vi "TSM DAQmx Relay Initialize Sessions.vi"(0 "TSM context":T1) -> (15 "error out":errorcluster)   [LabVIEW 2019]
doc: "Use this VI to initialize sessions for all NI 2567 Relay Driver Instruments in the pin map associated with the test program."
uses:
  <vilib>/NI_TestStand_SemiconductorModule/NI_TestStand_Semiconductor_Module.lvlibp/PinMap/General/SemiconductorModuleContext.ctl
  <vilib>/DAQmx/create/channels.llb/DAQmx Create Channel (DO-Digital Output).vi
  <vilib>/NI_TestStand_SemiconductorModule/NI_TestStand_Semiconductor_Module.lvlibp
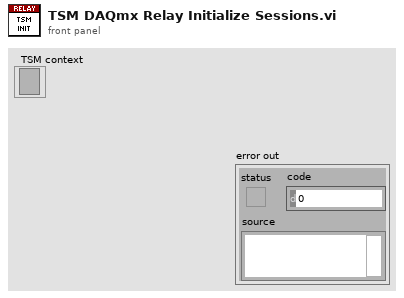
[diagram p1: front panel]
types:
  T1 = typedef "NI_TestStand_Semiconductor_Module.lvlibp/SemiconductorModuleContext.ctl" = refnum<k7>
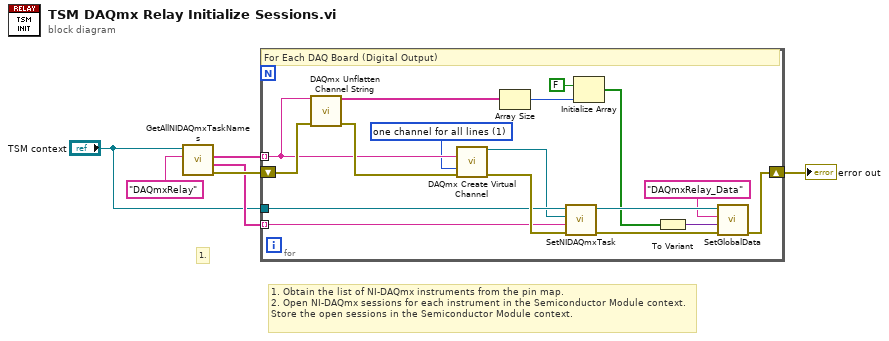
[diagram p0: block diagram]
diagram:
  # "1."
  # "1. Obtain the list of NI-DAQmx instruments from the pin map.\n2. Open NI-DAQmx sessions for each instrument in the Semiconductor Module context. Store the open sessions in the Semiconductor Module context."
  n1 = call <vilib>:"GetAllNIDAQmxTaskNames.vi"("Task Type"="DAQmxRelay", "Semiconductor Module Context"="TSM context") -> ("error out"=w6:errorcluster, "Task Names"=w3:string[], "Channel Lists"=w4:string[])  [unwired: 6 in, 1 out]
  n2 = for {
    tunnel: w4 -> [w10] mode=indexing
    shift-right: [w16] -> w1
    shift-left: w6 -> [w20]
    tunnel: w3 -> [w11] mode=indexing
    tunnel: "TSM context" -> [w22]
    w9 = 1 items=["one channel for each line", "one channel for all lines"] ("line grouping")
    # "For Each DAQ Board (Digital Output)"
    n3 = call <vilib>:"DAQmx Unflatten Channel String.vi"("names in"=w10, "error in"=w20) -> ("names out"=w18:string[], "error out"=w19:errorcluster)  [unwired: 12 in]
    n4 = call-poly <vilib>:"DAQmx Create Virtual Channel.vi"("lines"=w10, "line grouping"=w9, "error in"=w19) -> ("task out"=w21:refnum<k21>, "error out"=w23:errorcluster)  [unwired: 11 in]
    n5 = Array Size(array=w18) -> (size(s)=w14:i32)
    n6 = call <vilib>:"SetNIDAQmxTask.vi"("error in (no error)"=w23, "Task Name"=w11, "DAQmx Task"=w21, "Semiconductor Module Context"=w22) -> ("error out"=w17:errorcluster, "Semiconductor Module Context Out"=w13:T1)  [unwired: 6 in]
    n7 = Initialize Array(FALSE, w14) -> (w8:bool[])
    n8 = To Variant(anything=w8) -> (Variant=w7:variant)
    n9 = call <vilib>:"SetGlobalData.vi"("error in (no error)"=w17, "Data"=w7, "Data Id"="DAQmxRelay_Data", "Semiconductor Module Context"=w13) -> ("error out"=w16:errorcluster)  [unwired: 5 in, 1 out]
  }
  "error out" <- w1
